vi "to u64.vi"(11 "channel":T1) -> (3 "Numeric":u64)   [LabVIEW 2020]
types:
  T1 = cluster{"Real":fxp<+/-,16,3>, "Imag":fxp<+/-,16,3>}
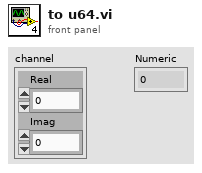
[diagram p1: front panel]
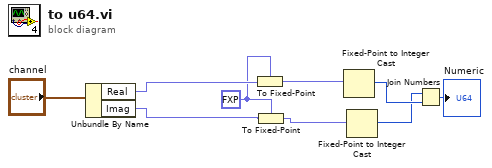
[diagram p0: block diagram]
diagram:
  w3 = fxp<+/-,32,11> 0.0 ("fixed-point type")
  n1 = Unbundle By Name("channel") -> ("Real"=w8:fxp<+/-,16,3>, "Imag"=w2:fxp<+/-,16,3>)
  n2 = To Fixed-Point(fixed-point type=w3, number=w8) -> (fixed-point=w4:fxp<+/-,32,11>)
  n3 = To Fixed-Point(fixed-point type=w3, number=w2) -> (fixed-point=w5:fxp<+/-,32,11>)
  n4 = Fixed-Point to Integer Cast(1:w4) -> (0:w7:i32)
  n5 = Fixed-Point to Integer Cast(1:w5) -> (0:w6:i32)
  n6 = Join Numbers(hi=w6, lo=w7) -> ((hi.lo)=→"Numeric":u64)
